vi "configuration UI.vi"() -> ()   [LabVIEW 2013, in "EthernetIP editor node.lvclass"]
uses:
  EthernetIP editor node.lvclass
  <vilib>/CEF_TreeControl/Node/NodeRef.ctl
  <vilib>/CEF_TreeControl/Node/NISE_CEF_Node.lvclass
  <vilib>/NI/AMC/Message Queue.ctl
  <vilib>/NI/AMC/Message.ctl
  <vilib>/NI/Tools/Keyed Array/KeyedArray.ctl
  <vilib>/CEF_TreeControl/Node/UserEventRef.ctl
  <vilib>/CEF_TreeControl/Controls/EventCluster.ctl
  <vilib>/NI/Module Execution Interface/Engine Configuration/engine configuration.lvclass
  <vilib>/NI/Tag Bus Data Framework/Configuration Editor/Classes/Engine Parent/Engine Parent Editor Node.lvclass
  <vilib>/NI/TBM Modules/Ethernet IP/configuration/EthernetIP configuration.lvclass
  <vilib>/NI/Tag Bus/tag/tag descriptor.lvclass
  <vilib>/NI/Tag Bus/tag/Data Type.ctl
  <vilib>/NI/Tag Bus/tag/tag descriptor.lvclass/tag descriptor.ctl
  EthernetIP editor node.lvclass/EthernetIP editor node.ctl
  <vilib>/NI/Tag Bus Module Framework/root configuration/TBM configuration.lvclass/TBM configuration.ctl
  <vilib>/NI/Tag Bus/tag/write tag name.vi
  <vilib>/NI/Tag Bus/tag/write data type.vi
  <vilib>/NI/Tag Bus Data Framework/Configuration Editor/Classes/Module editor node/Read Module Configuration.vi
  <vilib>/NI/Tag Bus Module Framework/root configuration/create GUID.vi
  <vilib>/NI/Tag Bus Module Framework/root configuration/TBM configuration.lvclass
  <vilib>/NI/Tag Bus Module Framework/module configuration/TBM module configuration.lvclass
  <vilib>/CEF_TreeControl/NISE_CEF_TreeControl.lvlib
  <vilib>/NI/Tag Bus Data Framework/Configuration Editor/Classes/Module editor node/module editor node.lvclass
  <vilib>/NI/Tools/Keyed Array/Tools_KeyedArray.lvlib
  <vilib>/NI/AMC/AMC.lvlib
panel:
  in  "Tab Control":enum32{"Assemblies", "Channels"}(tab)
  in  "Configure Assembly":bool
  in  "Remove Assembly":bool
  in  "Add Assembly":bool
  in  "assemblies":i32(listbox)
  in  "Remove Button":bool
  in  "Add Button":bool
  in  "channel":i32(listbox)
  in  "settings":bool
  in  "user event":T1
  in  "main queue":T2
  in  "node ref":T3
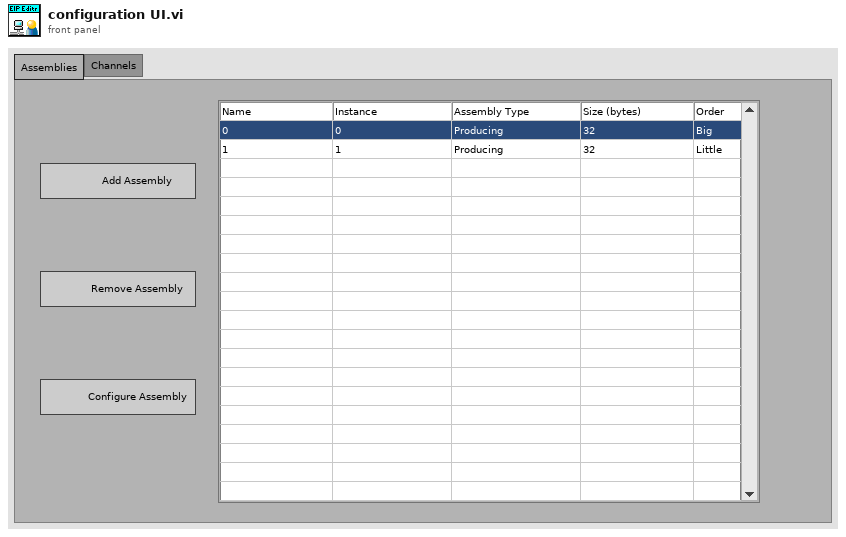
[diagram p1: front panel]
types:
  T1 = typedef "NISE_CEF_Node.lvclass/UserEventRef.ctl" = refnum<user-event>
  T2 = typedef "AMC.lvlib/Message Queue.ctl" = refnum<queue>
  T3 = typedef "NISE_CEF_Node.lvclass/NodeRef.ctl" = refnum<data-value>
  T4 = typedef "NISE_CEF_TreeControl.lvlib/EventCluster.ctl" = cluster{"command":string, "data":string}
  T5 = typedef "tag bus.lvlib/tag descriptor.lvclass/Data Type.ctl" = enum16{"Double", "Single", "I64", "I32", "I16", "I8", "U64", "U32", "U16", "U8", "Boolean", "String", "Array of Double", "Array of Single", "Array of I64", "Array of I32", "Array of I16", "Array of I8", "Array of U64", "Array of U32", "Array of U16", "Array of U8", "Array of Boolean", "Array of String"}
  T6 = typedef "EthernetIP editor node.lvclass/table line.ctl" = cluster{"eip channels":refnum<class "EthernetIP Channel.lvclass">, "tag name":string}
  T7 = typedef "LVPoint32TypeDef.ctl" = cluster{"Horizontal":i32, "Vertical":i32}
  T8 = typedef "LVRowAndColumnTypeDef.ctl" = cluster{"Row":i32, "Column":i32}
  T9 = typedef "EthernetIP configuration.lvclass/assembly definition.ctl" = cluster{"name":string, "Instance ID":u32, "Type":T10, "Size (bytes)":u32, "big endian?":bool}
  T10 = typedef "EthernetIP configuration.lvclass/assembly type.ctl" = enum32{"Producing", "Consuming"}
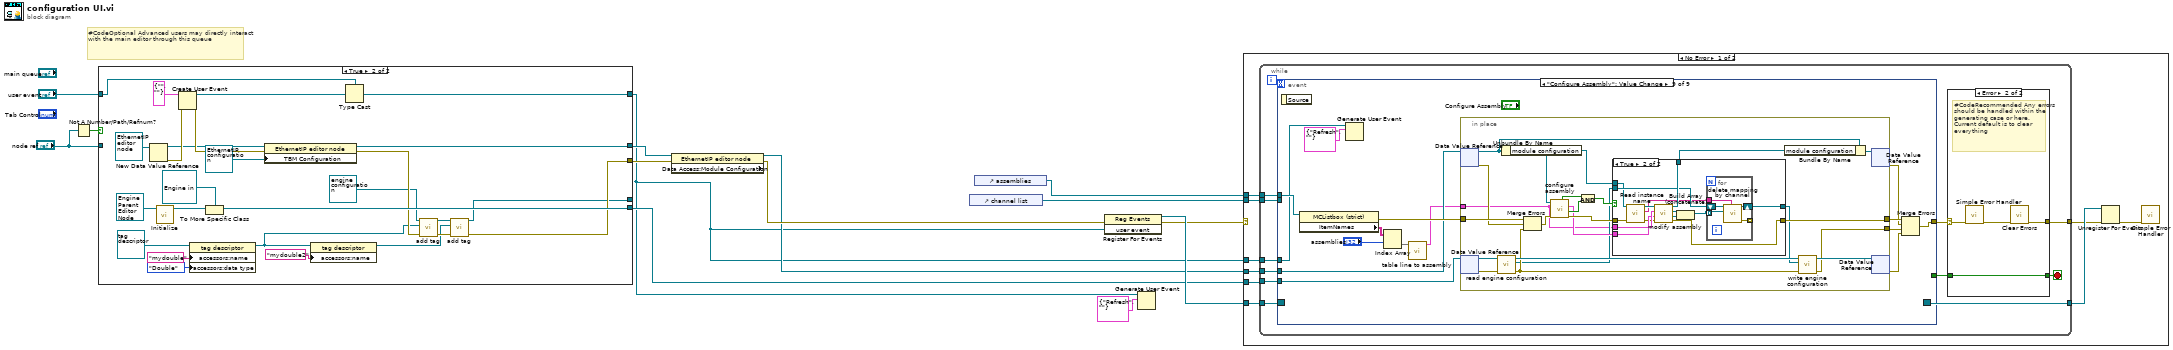
[diagram p0: block diagram]
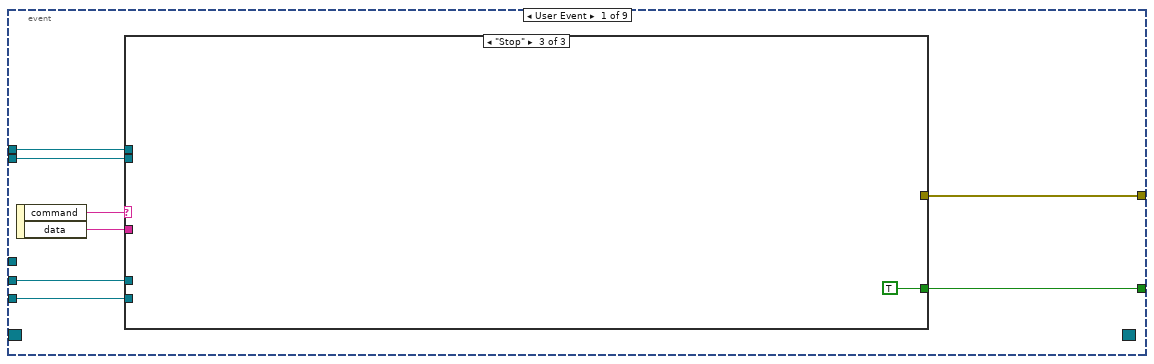
[diagram p3: hidden frame]
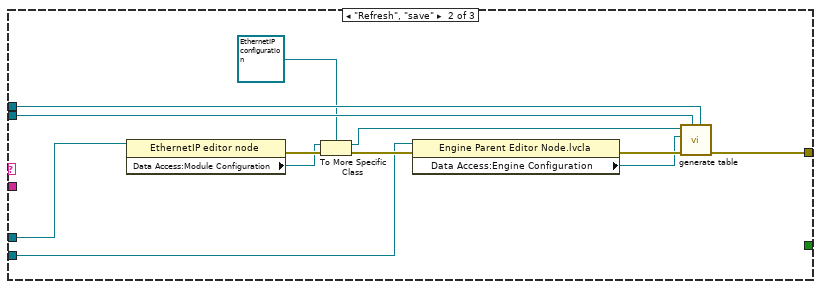
[diagram p5: hidden frame]
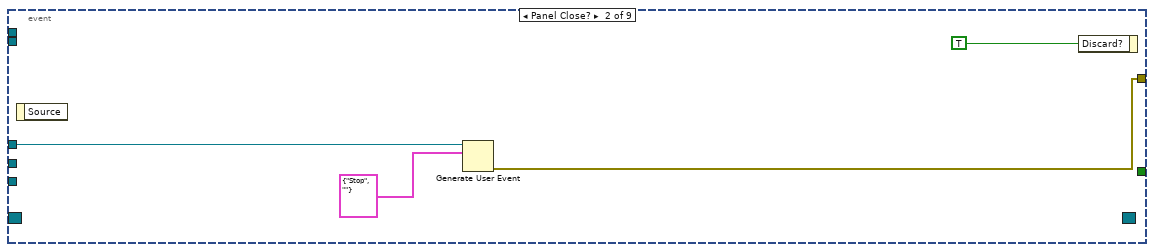
[diagram p6: hidden frame]
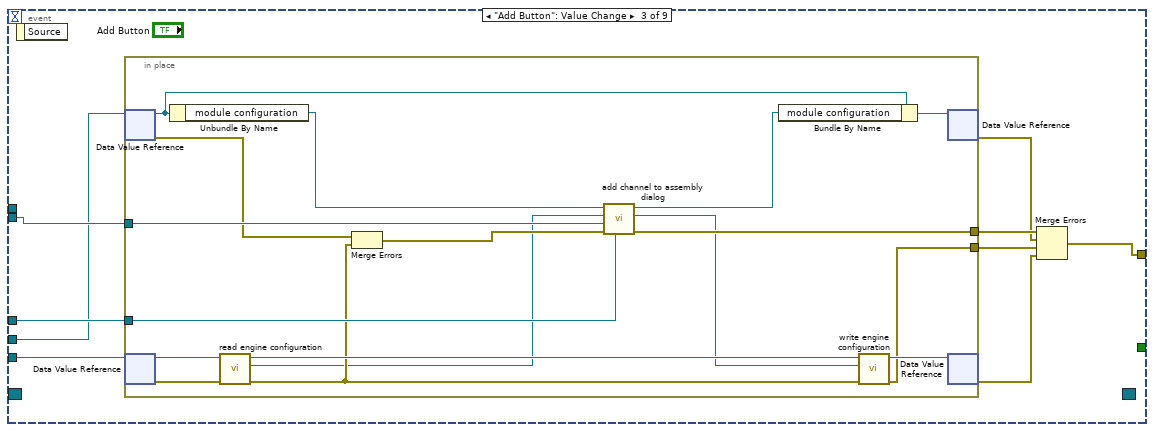
[diagram p7: hidden frame]
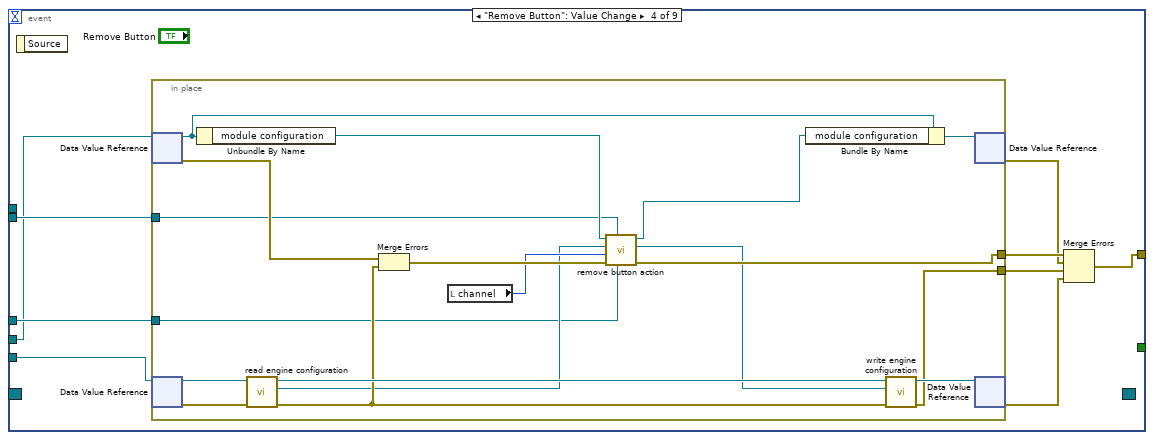
[diagram p8: hidden frame]
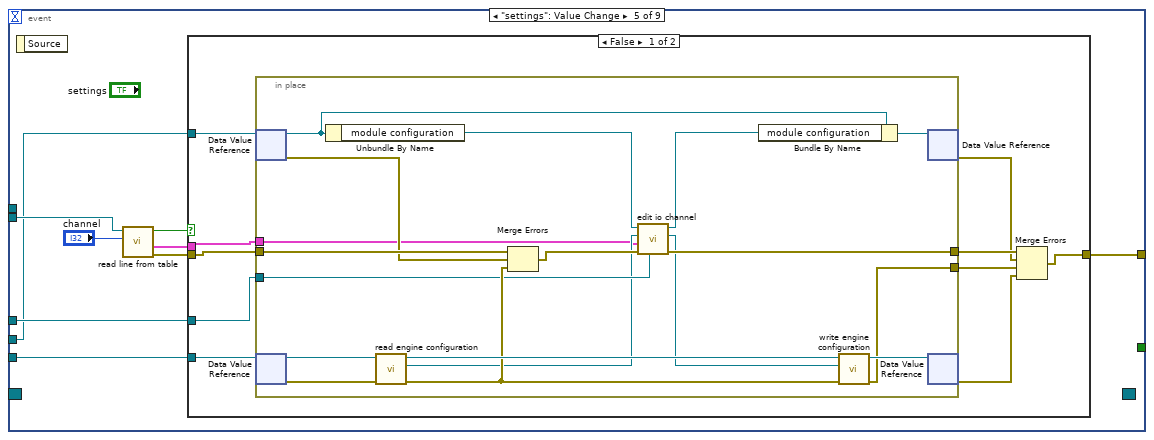
[diagram p9: hidden frame]
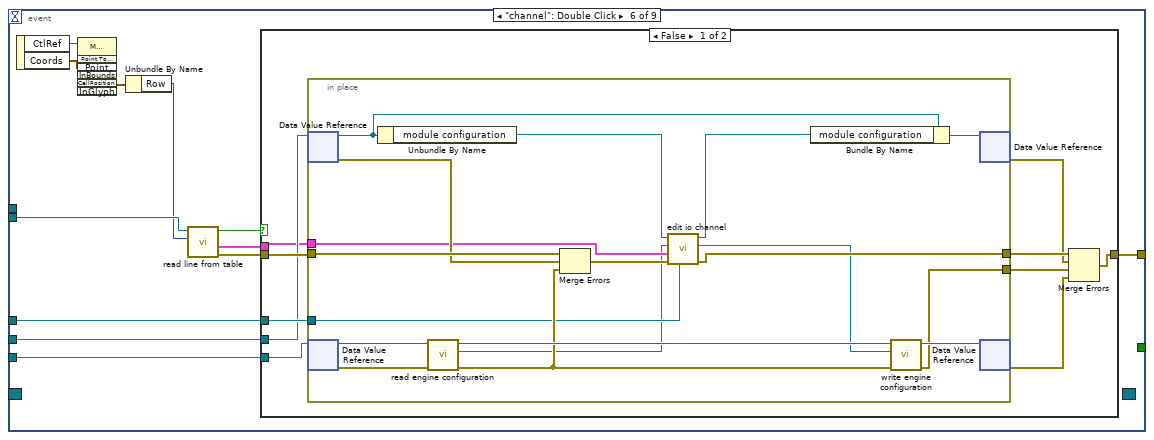
[diagram p11: hidden frame]
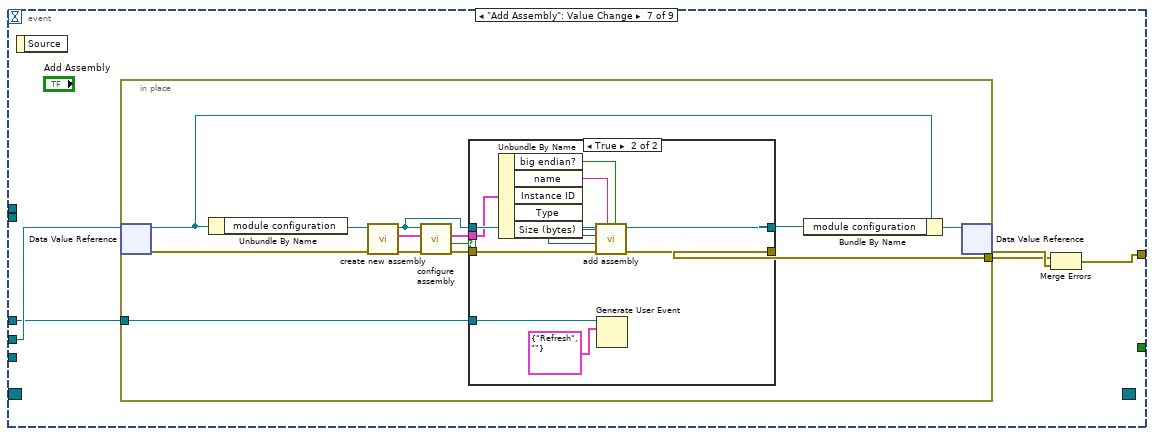
[diagram p13: hidden frame]
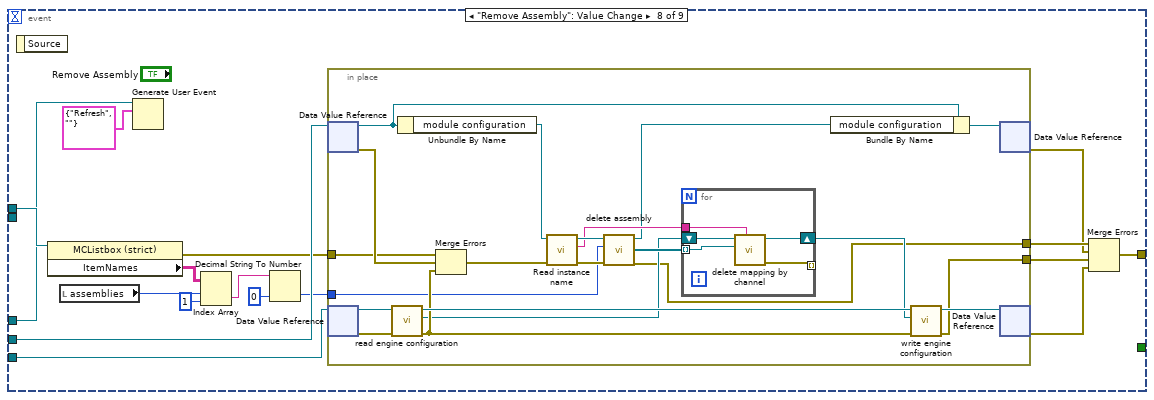
[diagram p15: hidden frame]
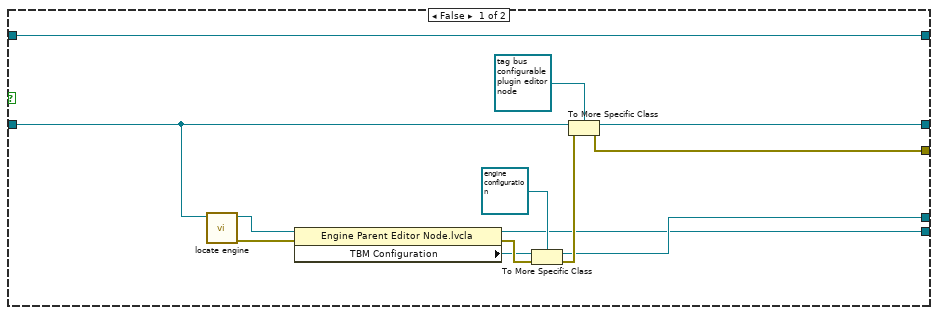
[diagram p18: hidden frame]
diagram:
  # "#CodeOptional Advanced users may directly interact with the main editor through this queue"
  n1 = Not A Number/Path/Refnum?(number/path/refnum="node ref") -> (NaN/Path/Refnum?=w12:bool)
  n2 = case shown="True" w12 {
    tunnel: "user event" -> [w27 w29]
    tunnel: [w27 w30] -> w2
    tunnel: "node ref" -> [w25 _]
    tunnel: [w24 w47] -> w8
    tunnel: [w23 w34] -> w10
    tunnel: [w16 w33] -> _
    tunnel: [w15 w44] -> w6
    frame False {
      n3 = call <vilib>:"locate engine.vi"("component"=w25) -> ("error out"=w20:errorcluster, "engine"=w22:refnum<data-value>)  [unwired: 9 in]
      n4 = property class="Engine Parent Editor Node.lvcla"(reference=w22, error in=w20) -> (reference out=w15:refnum<data-value>, error out=w19:errorcluster, "TBM Configuration"=w18:refnum<class "TBM configuration.lvclass">)
      n5 = To More Specific Class(target class=refnum<class "engine configuration.lvclass"> refnum ("engine configuration.lvclass"), reference=w18, error in=w19) -> (specific class reference=w16:refnum<class "engine configuration.lvclass">, error out=w17:errorcluster)
      n6 = To More Specific Class(target class=refnum<data-value> refnum ("data value reference"), reference=w25, error in=w17) -> (specific class reference=w24:refnum<data-value>, error out=w23:errorcluster)
    }
    frame True {
      n7 = New Data Value Reference(data value=refnum<class "EthernetIP editor node.lvclass"> refnum ("tag bus configurable plugin editor node")) -> (data value reference=w46:refnum<data-value>, error out=w49:errorcluster)  [unwired: 1 in]
      n8 = call-dynamic "Initialize.vi"("Engine in"=refnum<class "Engine Parent Editor Node.lvclass"> refnum) -> ("data value reference"=w45:T3)  [unwired: 8 in, 2 out]
      n9 = Create User Event(user event datatype=T4 {"command"="", "data"=""} ("event data"), error in=w49) -> (user event=w52:refnum<user-event>, error out=w48:errorcluster)
      n10 = property class="tag descriptor"(reference=refnum<class "tag descriptor.lvclass"> refnum ("tag descriptor"), "accessors:name"="mydouble" ("name"), "accessors:data type"=Data_Type."Double" ("data type")) -> (reference out=w31:refnum<class "tag descriptor.lvclass">)  [unwired: 1 in, 1 out]
      n11 = To More Specific Class(target class=refnum<data-value> refnum ("data value reference"), reference=w45) -> (specific class reference=w44:refnum<data-value>)  [unwired: 1 in, 1 out]
      n12 = property class="EthernetIP editor node"(reference=w46, error in=w48, "TBM Configuration"=refnum<class "EthernetIP configuration.lvclass"> refnum ("tag bus configurable plugin module configuration")) -> (reference out=w47:refnum<data-value>, error out=w38:errorcluster)
      n13 = property class="tag descriptor"(reference=w31, "accessors:name"="mydouble2" ("name")) -> (reference out=w32:refnum<class "tag descriptor.lvclass">)  [unwired: 1 in, 1 out]
      n14 = Type Cast(type=w29, x=w52) -> (*(type *) &x=w30:T1)
      n15 = call <vilib>:"add tag.vi"("error in"=w38, "tag descriptor"=w31, "engine configuration in"=refnum<class "engine configuration.lvclass"> refnum ("Engine Configuration")) -> ("error out"=w36:errorcluster, "engine configuration out"=w35:refnum<class "engine configuration.lvclass">)  [unwired: 7 in]
      n16 = call <vilib>:"add tag.vi"("error in"=w36, "tag descriptor"=w32, "engine configuration in"=w35) -> ("error out"=w34:errorcluster, "engine configuration out"=w33:refnum<class "engine configuration.lvclass">)  [unwired: 7 in]
    }
  }
  n17 = property class="EthernetIP editor node" props=["Data Access:Module Configuration"](reference=w8, error in=w10) -> (reference out=w7:refnum<data-value>, error out=w13:errorcluster)  [unwired: 1 out]
  n18 = control-ref of="channel list"() -> (w5:refnum<vi>)
  n19 = control-ref of="assemblies"() -> (w4:refnum<vi>)
  n20 = register-events(error in=w13, w2) -> (reference out=w14:refnum<event-registration>, error out=w1:errorcluster)  [unwired: 1 in]
  n21 = Generate User Event(user event=w2, event data cluster=T4 {"command"="Refresh", "data"=""} ("event data")) -> ()  [unwired: 2 in, 2 out]
  n22 = case shown="No Error" w1 {
    tunnel: w14 -> [w62 _]
    tunnel: w7 -> [w59 _]
    tunnel: w6 -> [w58 _]
    tunnel: w5 -> [w56 _]
    tunnel: w4 -> [w55 _]
    tunnel: w2 -> [w54 _]
    frame No Error {
      n23 = while {
        tunnel: w62 -> [w73]
        tunnel: [w72] -> w61
        tunnel: w59 -> [w68]
        tunnel: w58 -> [w67]
        tunnel: w54 -> [w66]
        tunnel: w56 -> [w64]
        tunnel: w55 -> [w63]
        tunnel: [w69] -> w60
        stop <- w71 stop-if-true
        n24 = event shown="[8] \"Configure Assembly\": Value Change" {
          selector: w73 -> [_ _ _ _ _ _ _ _ _]
          dyn-events: [_ _ _ _ _ _ _ _ _] -> w72
          timeout: _ -> [_ _ _ _ _ _ _ _ _]
          tunnel: [w87 _ _ _ _ _ _ _ _] -> w70
          tunnel: [w82 w101 w108 w135 w166 w207 w240 w273 w316] -> w65
          tunnel: w68 -> [w85 _ w110 w131 w158 w196 w239 w272 w313]
          tunnel: w67 -> [w84 _ w109 w132 w159 w197 _ w269 w314]
          tunnel: w66 -> [_ w103 w111 w133 w162 w204 w237 w278 w321]
          tunnel: w64 -> [w81 _ w112 w134 w160 w203 _ _ _]
          tunnel: w63 -> [w80 _ _ _ _ _ _ w285 w326]
          event User Event {
            n25 = event-data() -> ("command"=w86:string, "data"=w83:string)  [unwired: 1 in]
            n26 = case shown="\"Stop\"" w86 {
              tunnel: [_ _ TRUE] -> w87
              tunnel: w85 -> [_ w94 _]
              tunnel: w84 -> [_ w89 _]
              tunnel: w83 -> [_ _ _]
              tunnel: [_ w99 _] -> w82
              tunnel: w81 -> [_ w98 _]
              tunnel: w80 -> [_ w97 _]
              frame Default {
              }
              frame "Refresh", "save" {
                n27 = property class="EthernetIP editor node"(reference=w94) -> (error out=w95:errorcluster, "Data Access:Module Configuration"=w92:refnum<class "TBM module configuration.lvclass">)  [unwired: 1 in, 1 out]
                n28 = To More Specific Class(target class=refnum<class "EthernetIP configuration.lvclass"> refnum ("tag bus configurable plugin module configuration"), reference=w92, error in=w95) -> (specific class reference=w90:refnum<class "EthernetIP configuration.lvclass">, error out=w93:errorcluster)
                n29 = property class="Engine Parent Editor Node.lvcla"(reference=w89, error in=w93) -> (error out=w96:errorcluster, "Data Access:Engine Configuration"=w88:refnum<class "engine configuration.lvclass">)  [unwired: 1 out]
                n30 = call "generate table.vi"("assemblies"=w97, "table"=w98, "error in"=w96, "engine configuration in"=w88, "EthernetIP configuration in"=w90) -> ("error out"=w99:errorcluster)  [unwired: 6 in]
              }
              frame "Stop" {
              }
            }
          }
          event Panel Close? {
            n31 = event-data() -> ()  [unwired: 1 in, 1 out]
            n32 = Generate User Event(user event=w103, event data cluster=T4 {"command"="Stop", "data"=""} ("event data")) -> (error out=w101:errorcluster)  [unwired: 2 in, 1 out]
            n33 = event-data("Discard?"=TRUE) -> ()  [unwired: 1 in, 1 out]
          }
          event "Add Button": Value Change {
            n34 = event-data() -> ()  [unwired: 1 in, 1 out]
            n35 = in-place {
              in-place-border: [w130] -> w113
              in-place-border: w112 -> [w129]
              in-place-border: w111 -> [w128]
              in-place-border: [w120] -> w105
              n36 = in-place-dvr #1(w110) -> (w126:refnum<class "EthernetIP editor node.lvclass">, w122:errorcluster)
              n37 = in-place-dvr #2(w109) -> (w119:refnum<class "Engine Parent Editor Node.lvclass">, w118:errorcluster)
              n38 = Unbundle By Name(w126) -> ("module configuration"=w127:refnum<class "EthernetIP configuration.lvclass">)
              n39 = call <vilib>:"read engine configuration.vi"("error in"=w118, "Engine Parent Editor Node in"=w119) -> ("error out"=w116:errorcluster, "engine configuration"=w114:refnum<class "engine configuration.lvclass">, "Engine Parent Editor Node out"=w117:refnum<class "Engine Parent Editor Node.lvclass">)  [unwired: 7 in]
              n40 = Merge Errors(w122, w116) -> (w123:errorcluster)
              n41 = call "add channel to assembly dialog.vi"("user event"=w128, "error in"=w123, "channel list"=w129, "engine configuration in"=w114, "EthernetIP configuration in"=w127) -> ("error out"=w130:errorcluster, "engine configuration out"=w115:refnum<class "engine configuration.lvclass">, "EthernetIP configuration out"=w124:refnum<class "EthernetIP configuration.lvclass">)  [unwired: 4 in]
              n42 = Bundle By Name(cluster=w126, "module configuration"=w124) -> (w125:refnum<class "EthernetIP editor node.lvclass">)
              n43 = call <vilib>:"write engine configuration.vi"("error in"=w116, "engine configuration"=w115, "Engine Parent Editor Node in"=w117) -> ("error out"=w120:errorcluster, "Engine Parent Editor Node out"=w121:refnum<class "Engine Parent Editor Node.lvclass">)  [unwired: 7 in]
              n44 = in-place-dvr #1(w125) -> (w106:errorcluster)  [unwired: 1 out]
              n45 = in-place-dvr #2(w121) -> (w107:errorcluster)  [unwired: 1 out]
            }
            n46 = Merge Errors(w113, w106, w105, w107) -> (w108:errorcluster)
          }
          event "Remove Button": Value Change {
            n47 = event-data() -> ()  [unwired: 1 in, 1 out]
            n48 = in-place {
              in-place-border: [w147] -> w139
              in-place-border: [w153] -> w136
              in-place-border: w134 -> [w141]
              in-place-border: w133 -> [w140]
              n49 = in-place-dvr #3(w131) -> (w157:refnum<class "EthernetIP editor node.lvclass">, w155:errorcluster)
              n50 = in-place-dvr #4(w132) -> (w152:refnum<class "Engine Parent Editor Node.lvclass">, w151:errorcluster)
              n51 = Unbundle By Name(w157) -> ("module configuration"=w145:refnum<class "EthernetIP configuration.lvclass">)
              n52 = call <vilib>:"read engine configuration.vi"("error in"=w151, "Engine Parent Editor Node in"=w152) -> ("error out"=w149:errorcluster, "engine configuration"=w143:refnum<class "engine configuration.lvclass">, "Engine Parent Editor Node out"=w150:refnum<class "Engine Parent Editor Node.lvclass">)  [unwired: 7 in]
              n53 = Merge Errors(w155, w149) -> (w148:errorcluster)
              n54 = local read "channel"() -> (w144:i32)
              n55 = call "remove button action.vi"("user event"=w140, "channel list"=w141, "error in"=w148, "channel"=w144, "engine configuration in"=w143, "EthernetIP configuration in"=w145) -> ("error out"=w147:errorcluster, "engine configuration out"=w142:refnum<class "engine configuration.lvclass">, "EthernetIP configuration out"=w146:refnum<class "EthernetIP configuration.lvclass">)  [unwired: 3 in]
              n56 = Bundle By Name(cluster=w157, "module configuration"=w146) -> (w156:refnum<class "EthernetIP editor node.lvclass">)
              n57 = call <vilib>:"write engine configuration.vi"("error in"=w149, "engine configuration"=w142, "Engine Parent Editor Node in"=w150) -> ("error out"=w153:errorcluster, "Engine Parent Editor Node out"=w154:refnum<class "Engine Parent Editor Node.lvclass">)  [unwired: 7 in]
              n58 = in-place-dvr #3(w156) -> (w137:errorcluster)  [unwired: 1 out]
              n59 = in-place-dvr #4(w154) -> (w138:errorcluster)  [unwired: 1 out]
            }
            n60 = Merge Errors(w139, w137, w136, w138) -> (w135:errorcluster)
          }
          event "settings": Value Change {
            n61 = event-data() -> ()  [unwired: 1 in, 1 out]
            n62 = call "read line from table.vi"("line number"="channel", "channels table"=w160) -> ("error out"=w165:errorcluster, "line"=w164:T6, "empty channel?"=w161:bool)  [unwired: 6 in, 1 out]
            n63 = case shown="False" w161 {
              tunnel: [w171 w195] -> w166
              tunnel: w165 -> [w172 w195]
              tunnel: w164 -> [w167 _]
              tunnel: w162 -> [w170 _]
              tunnel: w159 -> [w169 _]
              tunnel: w158 -> [w168 _]
              frame False {
                n64 = in-place {
                  in-place-border: [w183] -> w176
                  in-place-border: w172 -> [w194]
                  in-place-border: [w189] -> w173
                  in-place-border: w170 -> [w182]
                  in-place-border: w167 -> [w177]
                  n65 = in-place-dvr #5(w168) -> (w193:refnum<class "EthernetIP editor node.lvclass">, w191:errorcluster)
                  n66 = in-place-dvr #6(w169) -> (w188:refnum<class "Engine Parent Editor Node.lvclass">, w187:errorcluster)
                  n67 = Unbundle By Name(w193) -> ("module configuration"=w181:refnum<class "EthernetIP configuration.lvclass">)
                  n68 = call <vilib>:"read engine configuration.vi"("error in"=w187, "Engine Parent Editor Node in"=w188) -> ("error out"=w185:errorcluster, "engine configuration"=w178:refnum<class "engine configuration.lvclass">, "Engine Parent Editor Node out"=w186:refnum<class "Engine Parent Editor Node.lvclass">)  [unwired: 7 in]
                  n69 = Merge Errors(w194, w191, w185) -> (w184:errorcluster)
                  n70 = call "edit io channel.vi"("user event"=w182, "error in"=w184, "line"=w177, "engine configuration in"=w178, "EthernetIP configuration in"=w181) -> ("error out"=w183:errorcluster, "engine configuration out"=w179:refnum<class "engine configuration.lvclass">, "EthernetIP configuration out"=w180:refnum<class "EthernetIP configuration.lvclass">)  [unwired: 4 in]
                  n71 = Bundle By Name(cluster=w193, "module configuration"=w180) -> (w192:refnum<class "EthernetIP editor node.lvclass">)
                  n72 = call <vilib>:"write engine configuration.vi"("error in"=w185, "engine configuration"=w179, "Engine Parent Editor Node in"=w186) -> ("error out"=w189:errorcluster, "Engine Parent Editor Node out"=w190:refnum<class "Engine Parent Editor Node.lvclass">)  [unwired: 7 in]
                  n73 = in-place-dvr #5(w192) -> (w174:errorcluster)  [unwired: 1 out]
                  n74 = in-place-dvr #6(w190) -> (w175:errorcluster)  [unwired: 1 out]
                }
                n75 = Merge Errors(w176, w174, w173, w175) -> (w171:errorcluster)
              }
              frame True {
              }
            }
          }
          event "channel": Double Click {
            n76 = event-data() -> ("CtlRef"=w202:refnum<vi>, "Coords"=w201:T7)  [unwired: 1 in]
            n77 = invoke class="MCListbox (strict)" method="Point To Row Column"(reference=w202, "Point"=w201) -> ("CellPosition"=w200:T8)  [unwired: 5 in, 6 out]
            n78 = Unbundle By Name(w200) -> ("Row"=w199:i32)
            n79 = call "read line from table.vi"("line number"=w199, "channels table"=w203) -> ("error out"=w206:errorcluster, "line"=w205:T6, "empty channel?"=w198:bool)  [unwired: 6 in, 1 out]
            n80 = case shown="False" w198 {
              tunnel: [w213 w236] -> w207
              tunnel: w206 -> [w212 w236]
              tunnel: w205 -> [w208 _]
              tunnel: w204 -> [w211 _]
              tunnel: w197 -> [w210 _]
              tunnel: w196 -> [w209 _]
              frame False {
                n81 = in-place {
                  in-place-border: [w224] -> w217
                  in-place-border: w212 -> [w235]
                  in-place-border: [w230] -> w214
                  in-place-border: w211 -> [w223]
                  in-place-border: w208 -> [w222]
                  n82 = in-place-dvr #7(w209) -> (w234:refnum<class "EthernetIP editor node.lvclass">, w232:errorcluster)
                  n83 = in-place-dvr #8(w210) -> (w229:refnum<class "Engine Parent Editor Node.lvclass">, w228:errorcluster)
                  n84 = Unbundle By Name(w234) -> ("module configuration"=w221:refnum<class "EthernetIP configuration.lvclass">)
                  n85 = call <vilib>:"read engine configuration.vi"("error in"=w228, "Engine Parent Editor Node in"=w229) -> ("error out"=w226:errorcluster, "engine configuration"=w218:refnum<class "engine configuration.lvclass">, "Engine Parent Editor Node out"=w227:refnum<class "Engine Parent Editor Node.lvclass">)  [unwired: 7 in]
                  n86 = Merge Errors(w235, w232, w226) -> (w225:errorcluster)
                  n87 = call "edit io channel.vi"("user event"=w223, "error in"=w225, "line"=w222, "engine configuration in"=w218, "EthernetIP configuration in"=w221) -> ("error out"=w224:errorcluster, "engine configuration out"=w219:refnum<class "engine configuration.lvclass">, "EthernetIP configuration out"=w220:refnum<class "EthernetIP configuration.lvclass">)  [unwired: 4 in]
                  n88 = Bundle By Name(cluster=w234, "module configuration"=w220) -> (w233:refnum<class "EthernetIP editor node.lvclass">)
                  n89 = call <vilib>:"write engine configuration.vi"("error in"=w226, "engine configuration"=w219, "Engine Parent Editor Node in"=w227) -> ("error out"=w230:errorcluster, "Engine Parent Editor Node out"=w231:refnum<class "Engine Parent Editor Node.lvclass">)  [unwired: 7 in]
                  n90 = in-place-dvr #7(w233) -> (w215:errorcluster)  [unwired: 1 out]
                  n91 = in-place-dvr #8(w231) -> (w216:errorcluster)  [unwired: 1 out]
                }
                n92 = Merge Errors(w217, w215, w214, w216) -> (w213:errorcluster)
              }
              frame True {
              }
            }
          }
          event "Add Assembly": Value Change {
            n93 = event-data() -> ()  [unwired: 1 in, 1 out]
            n94 = in-place {
              in-place-border: [w243] -> w238
              in-place-border: w237 -> [w242]
              n95 = in-place-dvr #9(w239) -> (w254:refnum<class "EthernetIP editor node.lvclass">, w246:errorcluster)
              n96 = Unbundle By Name(w254) -> ("module configuration"=w245:refnum<class "EthernetIP configuration.lvclass">)
              n97 = call "create new assembly.vi"("error in (no error)"=w246, "EthernetIP configuration in"=w245) -> ("error out"=w249:errorcluster, "assembly definition out"=w247:T9, "EthernetIP configuration out"=w248:refnum<class "EthernetIP configuration.lvclass">)  [unwired: 7 in]
              n98 = call "configure assembly.vi"("error in"=w249, "assembly definition in"=w247, "EthernetIP configuration"=w248) -> ("error out"=w252:errorcluster, "success"=w250:bool, "assembly definition out"=w251:T9)  [unwired: 5 in, 1 out]
              n99 = case shown="True" w250 {
                tunnel: w252 -> [w255 w268]
                tunnel: [w255 w267] -> w243
                tunnel: [w256 w266] -> w244
                tunnel: w248 -> [w256 w265]
                tunnel: w251 -> [_ w264]
                tunnel: w242 -> [_ w257]
                frame False {
                }
                frame True {
                  n100 = Unbundle By Name(w264) -> ("big endian?"=w259:bool, "name"=w260:string, "Instance ID"=w261:u32, "Type"=w262:T10, "Size (bytes)"=w263:u32)
                  n101 = call <vilib>:"add assembly.vi"("big endian?"=w259, "size (bytes)"=w263, "name"=w260, "error in"=w268, "Type"=w262, "instance ID"=w261, "EthernetIP configuration in"=w265) -> ("error out"=w267:errorcluster, "EthernetIP configuration out"=w266:refnum<class "EthernetIP configuration.lvclass">)  [unwired: 3 in]
                  n102 = Generate User Event(user event=w257, event data cluster=T4 {"command"="Refresh", "data"=""} ("event data")) -> ()  [unwired: 2 in, 2 out]
                }
              }
              n103 = Bundle By Name(cluster=w254, "module configuration"=w244) -> (w253:refnum<class "EthernetIP editor node.lvclass">)
              n104 = in-place-dvr #9(w253) -> (w241:errorcluster)  [unwired: 1 out]
            }
            n105 = Merge Errors(w238, w241) -> (w240:errorcluster)
          }
          event "Remove Assembly": Value Change {
            n106 = event-data() -> ()  [unwired: 1 in, 1 out]
            n107 = property class="MCListbox (strict)"(reference=w285) -> (error out=w270:errorcluster, "ItemNames"=w284:string[][])  [unwired: 1 in, 1 out]
            n108 = local read "assemblies"() -> (w283:i32)
            n109 = Generate User Event(user event=w278, event data cluster=T4 {"command"="Refresh", "data"=""} ("event data")) -> ()  [unwired: 2 in, 2 out]
            n110 = Index Array(array=w284, index (row)=w283, index (col)=1 ("disabled index (col)")) -> (element=w281:string)
            n111 = Decimal String To Number(string=w281, default (0L)=u32 0 ("default (0 I32)")) -> (number=w271:u32)  [unwired: 1 in, 1 out]
            n112 = in-place {
              in-place-border: [w287] -> w277
              in-place-border: [w302] -> w274
              in-place-border: w271 -> [w288]
              in-place-border: w270 -> [w297]
              n113 = in-place-dvr #10(w272) -> (w306:refnum<class "EthernetIP editor node.lvclass">, w304:errorcluster)
              n114 = in-place-dvr #11(w269) -> (w301:refnum<class "Engine Parent Editor Node.lvclass">, w300:errorcluster)
              n115 = call <vilib>:"read engine configuration.vi"("error in"=w300, "Engine Parent Editor Node in"=w301) -> ("error out"=w298:errorcluster, "engine configuration"=w290:refnum<class "engine configuration.lvclass">, "Engine Parent Editor Node out"=w299:refnum<class "Engine Parent Editor Node.lvclass">)  [unwired: 7 in]
              n116 = Unbundle By Name(w306) -> ("module configuration"=w291:refnum<class "EthernetIP configuration.lvclass">)
              n117 = Merge Errors(w297, w304, w298) -> (w292:errorcluster)
              n118 = call <vilib>:"Read instance name.vi"("error in"=w292, "configuration in"=w291) -> ("error out"=w295:errorcluster, "instance id"=w293:string, "configuration out"=w294:refnum<class "EthernetIP configuration.lvclass">)  [unwired: 7 in]
              n119 = call <vilib>:"delete assembly.vi"("error in"=w295, "instance ID"=w288, "EthernetIP configuration in"=w294) -> ("error out"=w287:errorcluster, "invalidated channelsu"=w296:refnum<class "EthernetIP Channel.lvclass">[], "EthernetIP configuration out"=w286:refnum<class "EthernetIP configuration.lvclass">)  [unwired: 6 in]
              n120 = for {
                shift-right: [w311] -> w289
                shift-left: w290 -> [w310]
                tunnel: w296 -> [w309] mode=indexing
                tunnel: [w308] -> _ mode=indexing
                tunnel: w293 -> [w307]
                n121 = call <vilib>:"delete mapping by channel.vi"("owner ID"=w307, "channel"=w309, "engine configuration in"=w310) -> ("error out"=w308:errorcluster, "engine configuration out"=w311:refnum<class "engine configuration.lvclass">)  [unwired: 7 in]
              }
              n122 = Bundle By Name(cluster=w306, "module configuration"=w286) -> (w305:refnum<class "EthernetIP editor node.lvclass">)
              n123 = call <vilib>:"write engine configuration.vi"("error in"=w298, "engine configuration"=w289, "Engine Parent Editor Node in"=w299) -> ("error out"=w302:errorcluster, "Engine Parent Editor Node out"=w303:refnum<class "Engine Parent Editor Node.lvclass">)  [unwired: 7 in]
              n124 = in-place-dvr #10(w305) -> (w275:errorcluster)  [unwired: 1 out]
              n125 = in-place-dvr #11(w303) -> (w276:errorcluster)  [unwired: 1 out]
            }
            n126 = Merge Errors(w277, w275, w274, w276) -> (w273:errorcluster)
          }
          event "Configure Assembly": Value Change {
            n127 = event-data() -> ()  [unwired: 1 in, 1 out]
            n128 = property class="MCListbox (strict)"(reference=w326) -> (error out=w315:errorcluster, "ItemNames"=w325:string[][])  [unwired: 1 in, 1 out]
            n129 = Generate User Event(user event=w321, event data cluster=T4 {"command"="Refresh", "data"=""} ("event data")) -> ()  [unwired: 2 in, 2 out]
            n130 = Index Array(array=w325, index (row)="assemblies") -> (element=w323:string[])  [unwired: 1 in]
            n131 = call "table line to assembly.vi"("ItemNames"=w323) -> ("assembly definition"=w312:T9)  [unwired: 10 in]
            n132 = in-place {
              in-place-border: [w333] -> w320
              in-place-border: w315 -> [w348]
              in-place-border: [w343] -> w317
              in-place-border: w312 -> [w327]
              n133 = in-place-dvr #12(w313) -> (w347:refnum<class "EthernetIP editor node.lvclass">, w345:errorcluster)
              n134 = in-place-dvr #13(w314) -> (w342:refnum<class "Engine Parent Editor Node.lvclass">, w341:errorcluster)
              n135 = call <vilib>:"read engine configuration.vi"("error in"=w341, "Engine Parent Editor Node in"=w342) -> ("error out"=w339:errorcluster, "engine configuration"=w328:refnum<class "engine configuration.lvclass">, "Engine Parent Editor Node out"=w340:refnum<class "Engine Parent Editor Node.lvclass">)  [unwired: 7 in]
              n136 = Unbundle By Name(w347) -> ("module configuration"=w329:refnum<class "EthernetIP configuration.lvclass">)
              n137 = Merge Errors(w348, w345, w339) -> (w330:errorcluster)
              n138 = call "configure assembly.vi"("error in"=w330, "assembly definition in"=w327, "EthernetIP configuration"=w329) -> ("error out"=w335:errorcluster, "success"=w338:bool, "assembly definition out"=w334:T9, "changed"=w337:bool)  [unwired: 5 in]
              n139 = And(x=w337, y=w338) -> (x .and. y?=w336:bool)
              n140 = case shown="True" w336 {
                tunnel: w335 -> [w351 w356]
                tunnel: [w351 w359] -> w333
                tunnel: w329 -> [w350 w352]
                tunnel: [w350 w365] -> w331
                tunnel: w327 -> [_ w364]
                tunnel: w334 -> [_ w363]
                tunnel: w328 -> [w349 w362]
                tunnel: [w349 w361] -> w332
                frame False {
                }
                frame True {
                  n141 = call <vilib>:"Read instance name.vi"("error in"=w356, "configuration in"=w352) -> ("error out"=w355:errorcluster, "instance id"=w353:string, "configuration out"=w354:refnum<class "EthernetIP configuration.lvclass">)  [unwired: 7 in]
                  n142 = call <vilib>:"modify assembly.vi"("error in"=w355, "new"=w363, "original"=w364, "EthernetIP configuration in"=w354) -> ("error out"=w359:errorcluster, "channel classification changed"=w357:refnum<class "EthernetIP Channel.lvclass">[], "invalidated channels"=w360:refnum<class "EthernetIP Channel.lvclass">[], "EthernetIP configuration out"=w365:refnum<class "EthernetIP configuration.lvclass">)  [unwired: 4 in]
                  n143 = Build Array (concatenate)(w360, w357) -> (w358:refnum<class "EthernetIP Channel.lvclass">[])
                  n144 = for {
                    shift-right: [w370] -> w361
                    shift-left: w362 -> [w369]
                    tunnel: w358 -> [w368] mode=indexing
                    tunnel: [w367] -> _ mode=indexing
                    tunnel: w353 -> [w366]
                    n145 = call <vilib>:"delete mapping by channel.vi"("owner ID"=w366, "channel"=w368, "engine configuration in"=w369) -> ("error out"=w367:errorcluster, "engine configuration out"=w370:refnum<class "engine configuration.lvclass">)  [unwired: 7 in]
                  }
                }
              }
              n146 = Bundle By Name(cluster=w347, "module configuration"=w331) -> (w346:refnum<class "EthernetIP editor node.lvclass">)
              n147 = call <vilib>:"write engine configuration.vi"("error in"=w339, "engine configuration"=w332, "Engine Parent Editor Node in"=w340) -> ("error out"=w343:errorcluster, "Engine Parent Editor Node out"=w344:refnum<class "Engine Parent Editor Node.lvclass">)  [unwired: 7 in]
              n148 = in-place-dvr #12(w346) -> (w318:errorcluster)  [unwired: 1 out]
              n149 = in-place-dvr #13(w344) -> (w319:errorcluster)  [unwired: 1 out]
            }
            n150 = Merge Errors(w320, w318, w317, w319) -> (w316:errorcluster)
          }
        }
        n151 = case shown="Error" w65 {
          selector: w65 -> [w74 w78]
          tunnel: [w75 w79] -> w71
          tunnel: w70 -> [w75 w79]
          tunnel: [w74 w76] -> w69
          frame No Error {
          }
          frame Error {
            # "#CodeRecommended Any errors should be handled within the generating case or here. Current default is to clear everything"
            n152 = call <vilib>:"Simple Error Handler.vi"("error in (no error)"=w78) -> ("error out"=w77:errorcluster)  [unwired: 4 in, 4 out]
            n153 = call <vilib>:"Clear Errors.vi"("error in (no error)"=w77) -> ("error out"=w76:errorcluster)  [unwired: 6 in]
          }
        }
      }
      n154 = Unregister For Events(event registration refnum=w61, error in=w60) -> (error out=w57:errorcluster)
      n155 = call <vilib>:"Simple Error Handler.vi"("error in (no error)"=w57) -> ()  [unwired: 4 in, 5 out]
    }
    frame Error {
    }
  }
